vi "Precise2.vi"() -> ()   [LabVIEW 2023]
uses:
  <vilib>/Platform/browser.llb/Open URL in Default Browser (path).vi
panel:
  out "error out":errorcluster
  in  "Log interval (ms)":dbl
  in  "Start logging":bool caption="Blank Button"
  in  "Open log folder":bool caption="Blank Button"
  out "Log file":string
  out "Temperature":T1(graph)
  out "Pressure":T1(graph)
  in  "Ids, (comma delimited)":string
  in  "USB port":refnum<visa-resource-name>
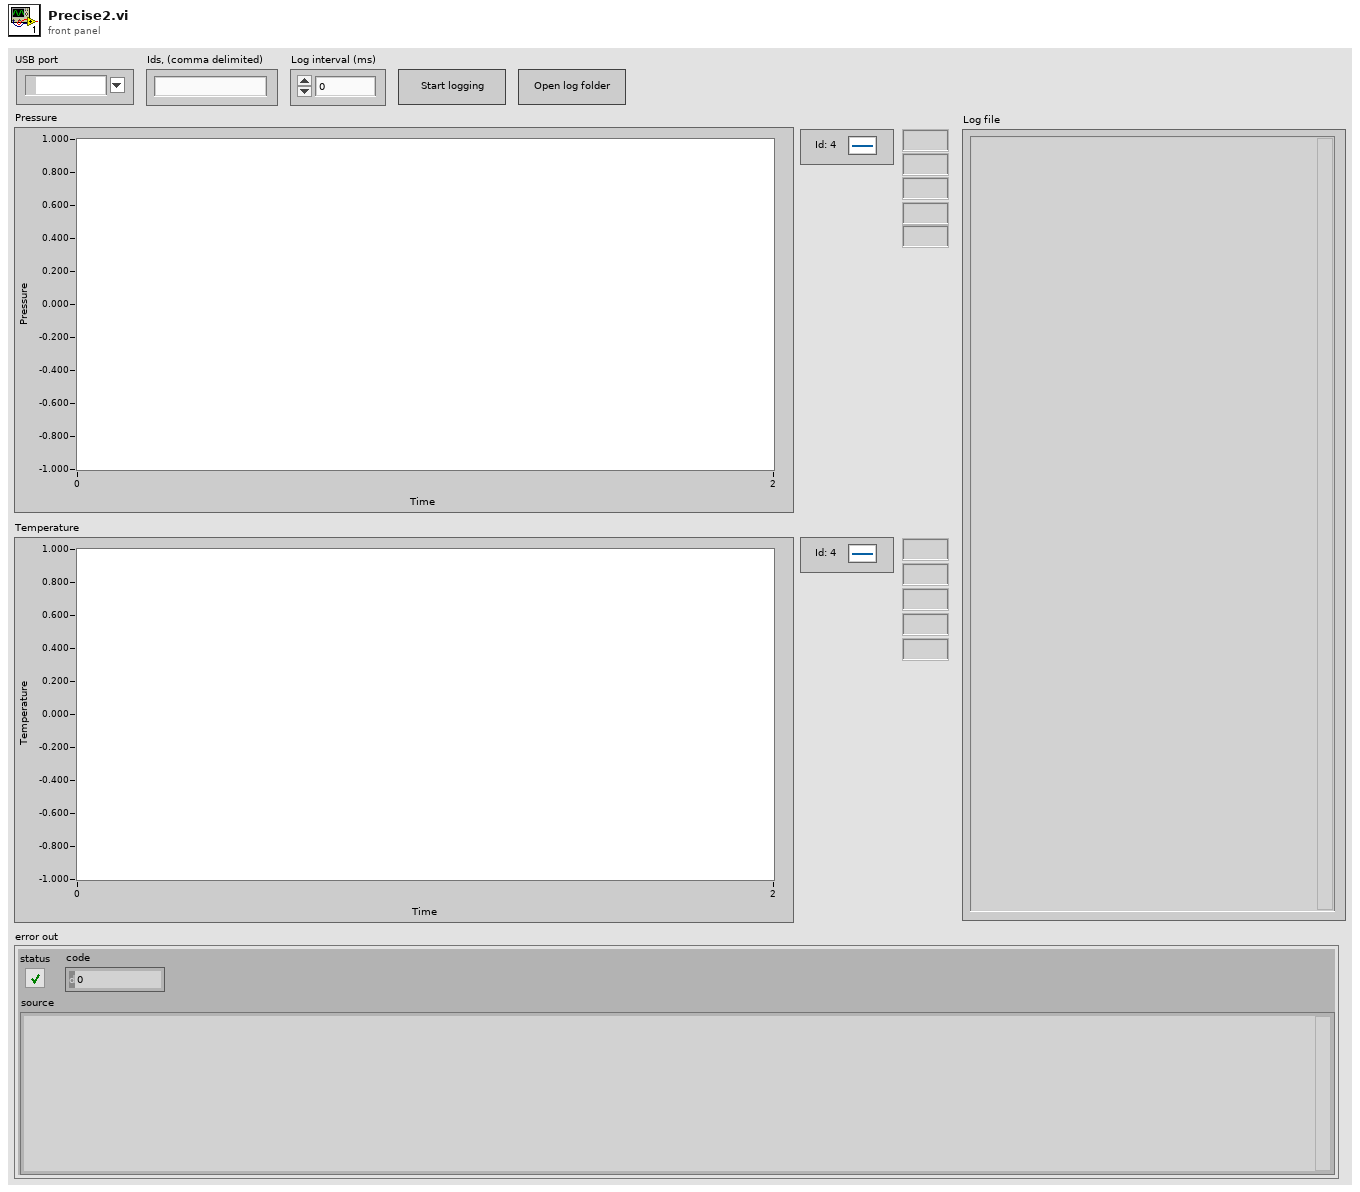
[diagram p1: front panel]
types:
  T1 = cluster{"[0]":dbl, "[1]":dbl, "[2]":dbl, "[3]":dbl, "[4]":dbl}
  T2 = cluster{"[0]":sgl, "[1]":sgl, "[2]":sgl, "[3]":sgl, "[4]":sgl}[]
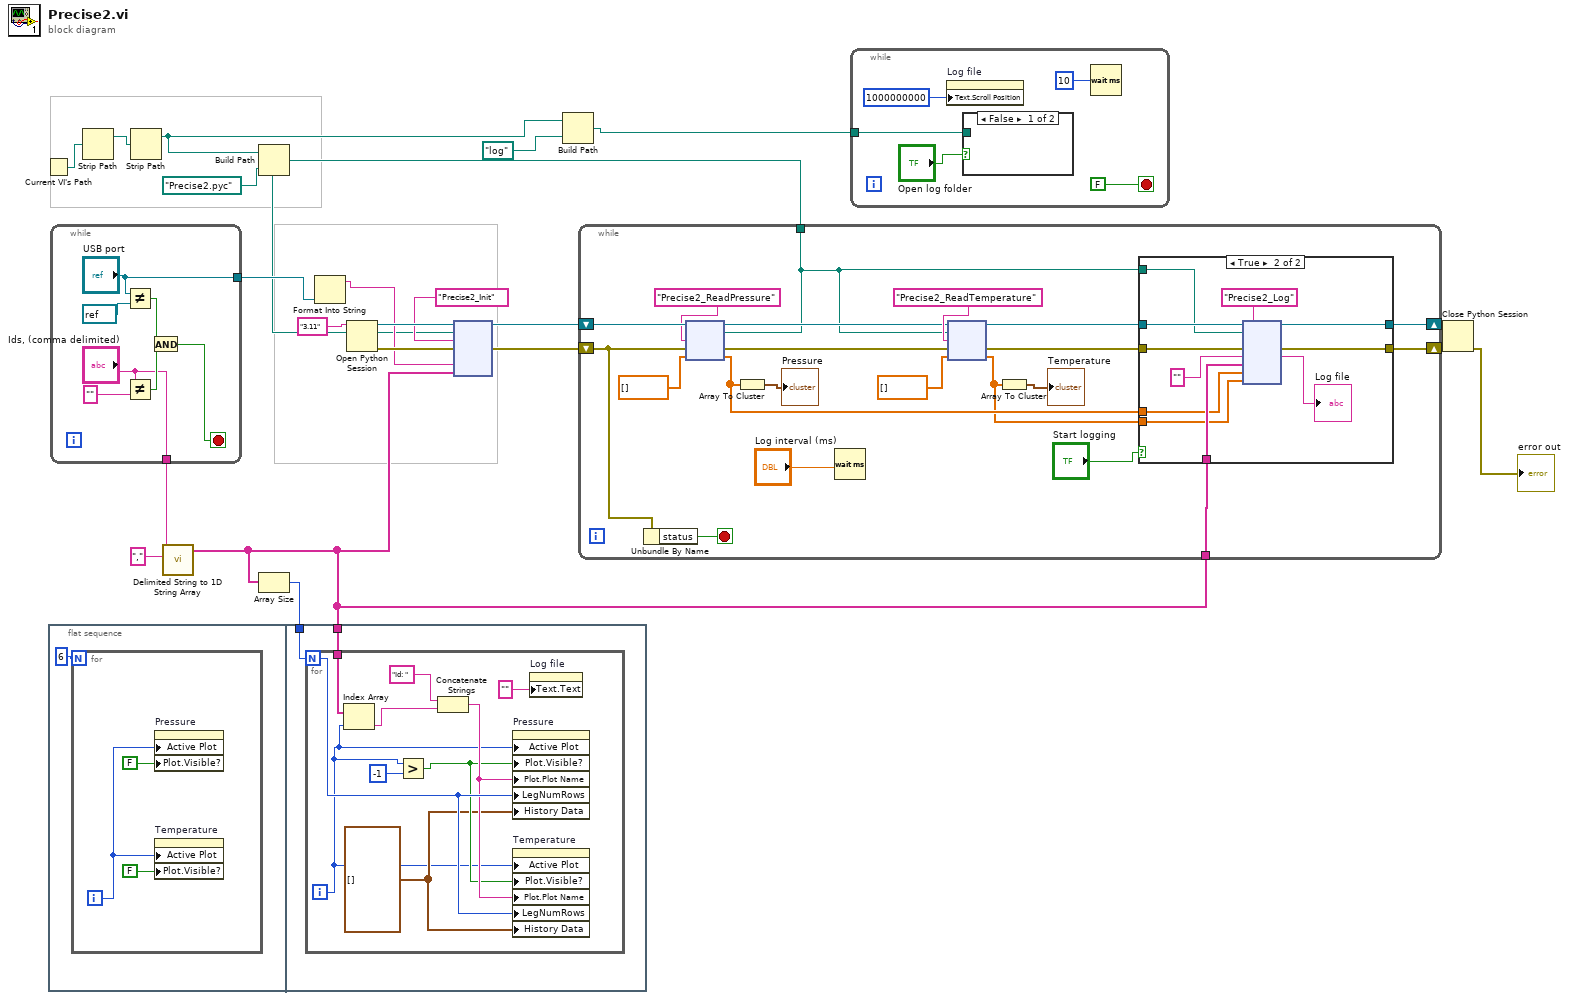
[diagram p0: block diagram]
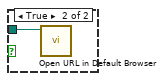
[diagram p2: hidden frame]
diagram:
  n1 = Current VI's Path() -> (path=w2:path)
  n2 = flat-sequence {
    tunnel: w9 -> [w28]
    tunnel: w7 -> [w27]
    frame #0 {
      n3 = for {
        N: 6 -> [_]
        i -> [w26]
        n4 = property on="Pressure" class="WFChart (strict)"("Active Plot"=w26, "Plot.Visible?"=FALSE ("Plot.Visible")) -> ()  [unwired: 2 in, 2 out]
        n5 = property on="Temperature" class="WFChart (strict)"("Active Plot"=w26, "Plot.Visible?"=FALSE ("Plot.Visible")) -> ()  [unwired: 2 in, 2 out]
      }
    }
    frame #1 {
      n6 = for {
        N: w28 -> [w37]
        tunnel: w27 -> [w31]
        i -> [w30]
        w32 = T2 [] ("History Data")
        n7 = Index Array(array=w31, index=w30) -> (element=w29:string)
        n8 = Greater?(x=w30, y=-1) -> (0:w34:bool)
        n9 = Concatenate Strings("Id: " ("string"), w29) -> (w36:string)
        n10 = property on="Pressure" class="WFChart (strict)"("Active Plot"=w30, "Plot.Visible?"=w34, "Plot.Plot Name"=w36, "LegNumRows"=w37, "History Data"=w32) -> ()  [unwired: 2 in, 2 out]
        n11 = property on="Temperature" class="WFChart (strict)"("Active Plot"=w30, "Plot.Visible?"=w34, "Plot.Plot Name"=w36, "LegNumRows"=w37, "History Data"=w32) -> ()  [unwired: 2 in, 2 out]
        n12 = property on="Log file" class="Str"("Text.Text"="") -> ()  [unwired: 2 in, 2 out]
      }
    }
  }
  n13 = while {
    tunnel: ["USB port"] -> w15
    tunnel: ["Ids, (comma delimited)"] -> w11
    stop <- w39 stop-if-true
    n14 = Not Equal?(x="USB port", y=refnum<visa-resource-name> refnum) -> (x != y?=w43:bool)
    n15 = Not Equal?(x="Ids, (comma delimited)", y="") -> (x != y?=w42:bool)
    n16 = And(x=w43, y=w42) -> (x .and. y?=w39:bool)
  }
  n17 = Strip Path(path=w2) -> (stripped path=w3:path)  [unwired: 1 out]
  n18 = Strip Path(path=w3) -> (stripped path=w4:path)  [unwired: 1 out]
  n19 = call <vilib>:"Delimited String to 1D String Array.vi"("delimiter"=",", "delimited string"=w11) -> ("string array"=w7:string[])  [unwired: 9 in]
  n20 = Build Path(base path=w4, name or relative path=path "Precise2.pyc") -> (appended path=w1:path)
  n21 = Array Size(array=w7) -> (size(s)=w9:i32)
  n22 = Format Into String(w15) -> (resulting string=w14:string)  [unwired: 3 in, 1 out]
  n23 = Open Python Session(python version="3.11" ("Python version")) -> (session out=w20:refnum<k35>, error out=w19:errorcluster)  [unwired: 2 in]
  n24 = node(w20, w1, "Precise2_Init" ("function name"), w19, w14, w7) -> (w13:refnum<k35>, w12:errorcluster)  [unwired: 4 in, 2 out]
  n25 = Build Path(base path=w4, name or relative path=path "log") -> (appended path=w6:path)
  n26 = while {
    shift-right: [w54] -> w22
    shift-left: w13 -> [w66]
    shift-right: [w52] -> w21
    shift-left: w12 -> [w62]
    tunnel: w1 -> [w50]
    tunnel: w7 -> [w49]
    stop <- w61 stop-if-true
    n27 = Unbundle By Name(w62) -> ("status"=w61:bool)
    n28 = node(w66, w50, "Precise2_ReadPressure" ("function name"), w62, dbl[] []) -> (w58:refnum<k35>, w57:errorcluster, w48:dbl[])  [unwired: 2 out]
    n29 = Array To Cluster(array=w48) -> (cluster=→"Pressure":T1)
    n30 = Wait (ms)(milliseconds to wait="Log interval (ms)") -> ()  [unwired: 1 out]
    n31 = node(w58, w50, "Precise2_ReadTemperature" ("function name"), w57, dbl[] []) -> (w53:refnum<k35>, w51:errorcluster, w47:dbl[])  [unwired: 2 out]
    n32 = Array To Cluster(array=w47) -> (cluster=→"Temperature":T1)
    n33 = case shown="True" "Start logging" {
      tunnel: [w68 w78] -> w54
      tunnel: w53 -> [w68 w79]
      tunnel: [w67 w76] -> w52
      tunnel: w51 -> [w67 w77]
      tunnel: w50 -> [_ w75]
      tunnel: w49 -> [_ w73]
      tunnel: w48 -> [_ w72]
      tunnel: w47 -> [_ w71]
      frame False {
      }
      frame True {
        n34 = node(w79, w75, "Precise2_Log" ("function name"), w77, "", w73, w72, w71) -> (w78:refnum<k35>, w76:errorcluster, →"Log file":string)  [unwired: 3 in, 2 out]
      }
    }
  }
  n35 = while {
    tunnel: w6 -> [w83]
    stop <- FALSE stop-if-true
    n36 = property on="Log file" class="Str"("Text.Scroll Position"=u32 1000000000) -> ()  [unwired: 2 in, 2 out]
    n37 = case shown="False" "Open log folder" {
      tunnel: w83 -> [_ w85]
      frame False {
      }
      frame True {
        n38 = call-poly <vilib>:"Open URL in Default Browser.vi"("path"=w85) -> ()  [unwired: 5 in, 2 out]
      }
    }
    n39 = Wait (ms)(milliseconds to wait=u32 10) -> ()  [unwired: 1 out]
  }
  n40 = Close Python Session(session in=w22, error in=w21) -> (11:→"error out":errorcluster)
